vi "запись.vi"() -> ()   [LabVIEW 2017]
uses:
  <vilib>/Utility/file.llb/Write Delimited Spreadsheet (DBL).vi
panel:
  in  "file path (dialog if empty)":path
  out "Waveform Graph":dbl[][](graph)
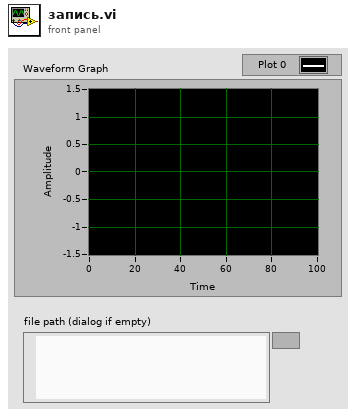
[diagram p1: front panel]
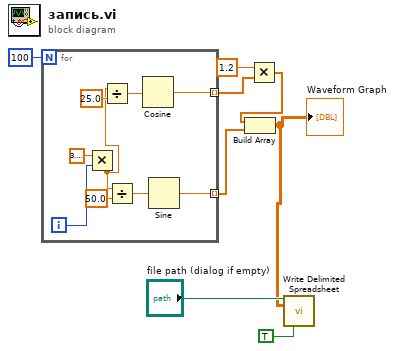
[diagram p0: block diagram]
diagram:
  n1 = for {
    N: 100 -> [_]
    tunnel: [w10] -> w5 mode=indexing
    tunnel: [w9] -> w7 mode=indexing
    i -> [w16]
    n2 = Multiply(x=3.141592653589793, y=w16) -> (x*y=w13:dbl)
    n3 = Divide(x=w13, y=25.0) -> (x/y=w11:dbl)
    n4 = Divide(x=w13, y=50.0) -> (x/y=w12:dbl)
    n5 = Cosine(x=w11) -> (cos(x)=w10:dbl)
    n6 = Sine(x=w12) -> (sin(x)=w9:dbl)
  }
  n7 = Multiply(x=1.2, y=w5) -> (x*y=w4:dbl[])
  n8 = Build Array(w4, w7) -> (w2:dbl[][])
  "Waveform Graph" <- w2
  n9 = call-poly <vilib>:"Write Delimited Spreadsheet.vi"("file path (dialog if empty)"="file path (dialog if empty)", "2D data"=w2, "transpose? (no:F)"=TRUE) -> ()  [unwired: 11 in, 2 out]
